vi "Init.vi"(8 "error in (no error)":errorcluster, 10 "Scene Item ID":i32, 11 "Scene Name":string) -> (0 "error out":errorcluster, 3 "GetSceneItemEnabled out":refnum<class "GetSceneItemEnabled.lvclass">)   [LabVIEW 2022 SP3, in "obs-websocket-lv.lvlib" / "GetSceneItemEnabled.lvclass"]
uses:
  GetSceneItemEnabled.lvclass
  GetSceneItemEnabled.lvclass/GetSceneItemEnabled.ctl
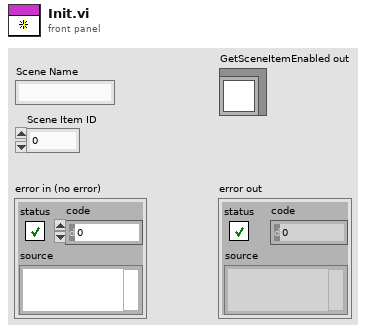
[diagram p1: front panel]
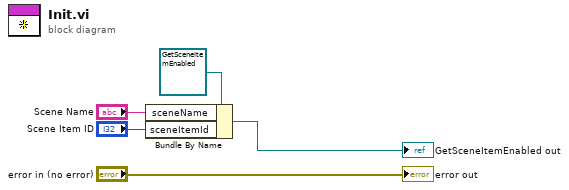
[diagram p0: block diagram]
diagram:
  n1 = Bundle By Name(cluster=refnum<class "GetSceneItemEnabled.lvclass"> refnum ("GetSceneItemEnabled in"), "sceneName"="Scene Name", "sceneItemId"="Scene Item ID") -> (→"GetSceneItemEnabled out":refnum<class "GetSceneItemEnabled.lvclass">)
  "error out" <- "error in (no error)"
